vi "decodeCamerasReferee.vi"(7 "previous VSS_Ref":T1={"FoulQuadrantVSS"=enum."NO_QUADRANT", "TeamColorVSS"=enum."NONE", "HalfVSS"=enum."SECOND_HALF", "Foul"=enum."GAME_ON", "timestamp"=0.0}, 8 "error in (no error)":errorcluster, 9 "RX":bool, 10 "element":u8[](array[numeric]), 11 "Vision in":refnum<class "Vision.lvclass">) -> (0 "error out":errorcluster, 1 "VSS_Ref":T1={"FoulQuadrantVSS"=enum."NO_QUADRANT", "TeamColorVSS"=enum."NONE", "HalfVSS"=enum."SECOND_HALF", "Foul"=enum."GAME_ON", "timestamp"=0.0}, 2 "SSL Game Status":T6, 3 "Vision out":refnum<class "Vision.lvclass">)   [LabVIEW 2023, in "Vision.lvclass"]
uses:
  Vision.lvclass
  Old vision/Controls/SSL Referee.ctl
  Old vision/Decode SSL and Refree Wrapper Package Folder/SSL Referee Team Info.ctl
  Referee_class/VSS_Ref.ctl
  Referee_class/Quadrant.ctl
  Referee_class/Color.ctl
  Referee_class/Halfs.ctl
  Referee_class/commands.ctl
  Referee_class/Referee.lvclass
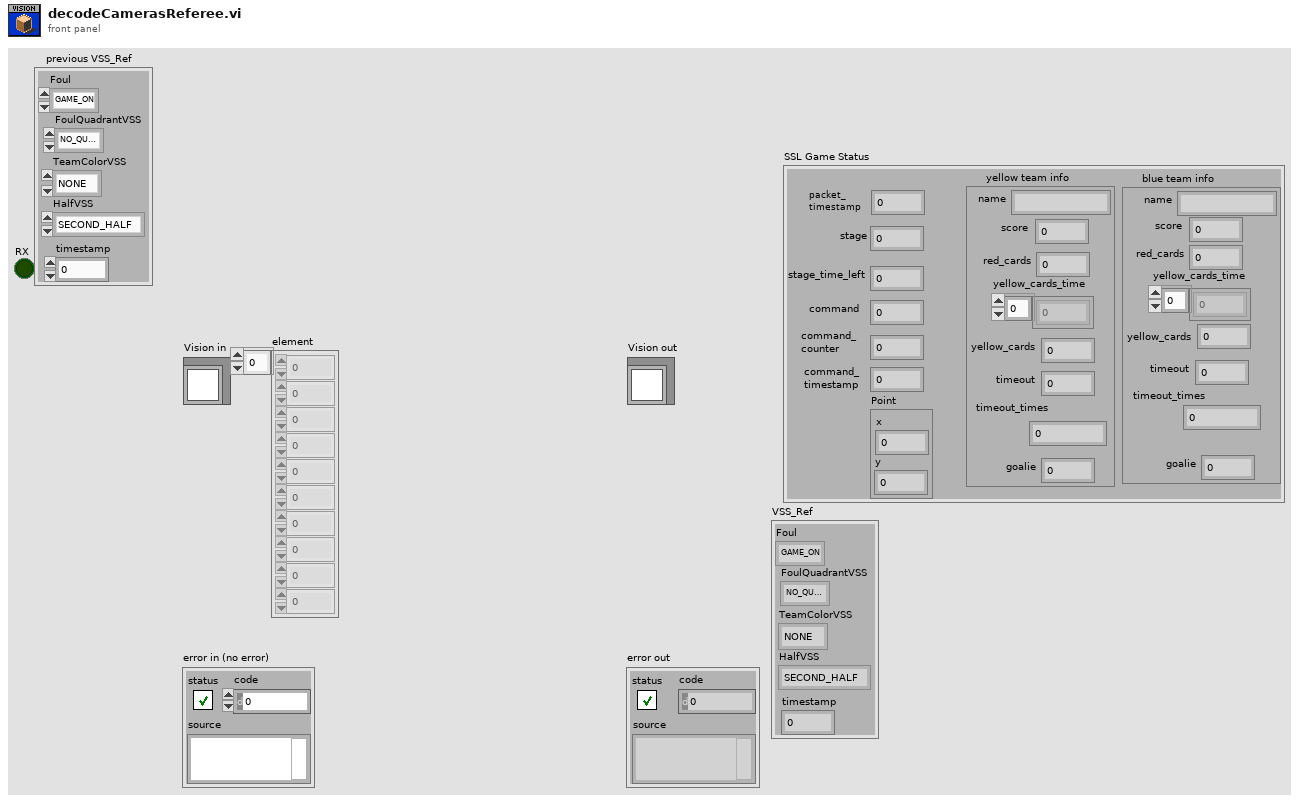
[diagram p1: front panel]
types:
  T1 = typedef "Referee.lvclass/VSS_Ref.ctl" = cluster{"FoulQuadrantVSS":T2, "TeamColorVSS":T3, "HalfVSS":T4, "Foul":T5, "timestamp":dbl}
  T2 = typedef "Quadrant.ctl" = enum16{"NO_QUADRANT", "QUADRANT_1", "QUADRANT_2", "QUADRANT_3", "QUADRANT_4"}
  T3 = typedef "Color.ctl" = enum16{"BLUE", "YELLOW", "NONE"}
  T4 = typedef "Halfs.ctl" = enum16{"NO_HALF", "FIRST_HALF", "SECOND_HALF", "OVERTIME_FIRST_HALF", "OVERTIME_SECOND_HALF", "PENALTY_SHOOTOUS"}
  T5 = typedef "Referee.lvclass/commands.ctl" = enum16{"FREE_KICK", "PENALTY_KICK", "GOAL_KICK", "FREE_BALL", "KICKOFF", "STOP", "GAME_ON", "HALT"}
  T6 = typedef "SSL Referee.ctl" = cluster{"packet_\ntimestamp":u64, "stage":u64, "stage_time_left":i32, "command ":u64, "command_\ncounter ":u32, "command_\ntimestamp":u64, "yellow team info":T7, "blue team info":T7, "Point":cluster{"x":sgl, "y":sgl}}
  T7 = typedef "SSL Referee Team Info.ctl" = cluster{"name":string, "score":u32, "red_cards":u32, "yellow_cards_time":u32[], "yellow_cards":u32, "timeout":u32, "timeout_times":u32, "goalie":u32}
  T8 = cluster{"Varint":u32, "Varint":u32, "Varint":u32, "Double":dbl, "Varint":u32}
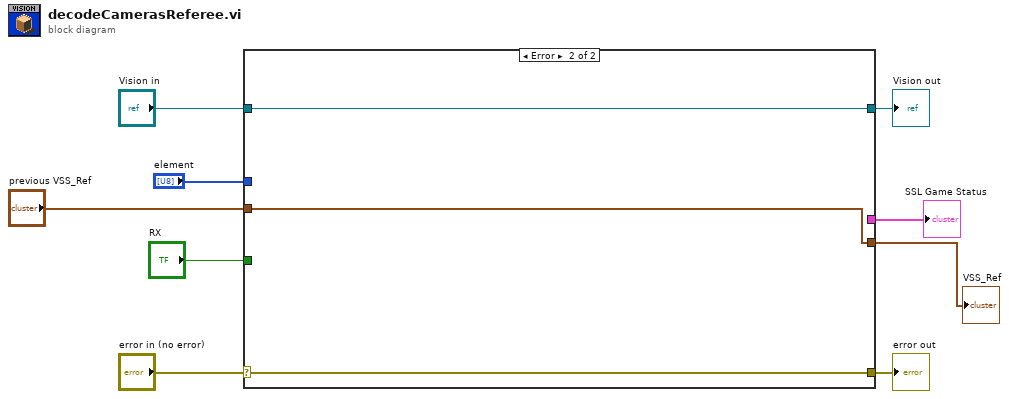
[diagram p0: block diagram]
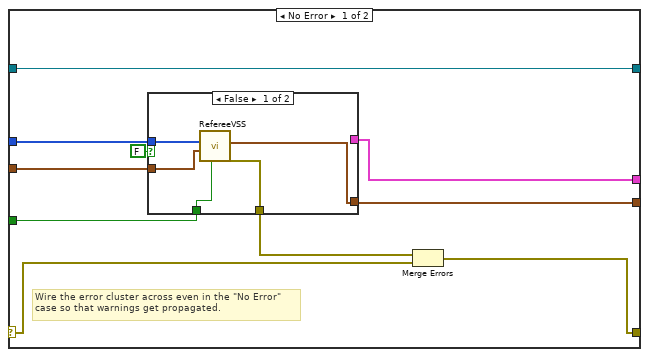
[diagram p2: hidden frame]
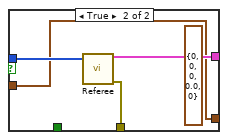
[diagram p3: hidden frame]
diagram:
  n1 = case shown="Error" "error in (no error)" {
    selector: "error in (no error)" -> [w15 w31]
    tunnel: [w14 w31] -> w8
    tunnel: [w19 w30] -> w6
    tunnel: "Vision in" -> [w19 w30]
    tunnel: "element" -> [w18 _]
    tunnel: [w17 _] -> w4
    tunnel: "RX" -> [w13 _]
    tunnel: [w11 w29] -> w2
    tunnel: "previous VSS_Ref" -> [w10 w29]
    frame No Error {
      # "Wire the error cluster across even in the \"No Error\"\ncase so that warnings get propagated."
      n2 = case shown="False" FALSE {
        tunnel: w18 -> [w22 w28]
        tunnel: [_ w27] -> w17
        tunnel: [w24 w26] -> w16
        tunnel: w13 -> [w23 _]
        tunnel: [w21 w25] -> w11
        tunnel: w10 -> [w20 w25]
        frame False {
          n3 = call "RefereeVSS.vi"("RX"=w23, "previous VSS_Ref 2"=w20, "element"=w22) -> ("error out 2"=w24:errorcluster, "VSS_Ref"=w21:T1)  [unwired: 7 in]
        }
        frame True {
          (unwired) T8 {"Varint"=0, "Varint"=0, "Varint"=0, "Double"=0.0, "Varint"=0} ("Cluster")
          n4 = call "Referee.vi"("element"=w28) -> ("output cluster"=w27:T6, "error out"=w26:errorcluster)  [unwired: 13 in]
        }
      }
      n5 = Merge Errors(w16, w15) -> (w14:errorcluster)
    }
    frame Error {
    }
  }
  "error out" <- w8
  "Vision out" <- w6
  "SSL Game Status" <- w4
  "VSS_Ref" <- w2
